vi "sub_dt_fgv.vi"(7 "cmd":enum16{"ini", "dt"}(ring)) -> (3 "dt":u32)   [LabVIEW 2018]
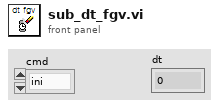
[diagram p1: front panel]
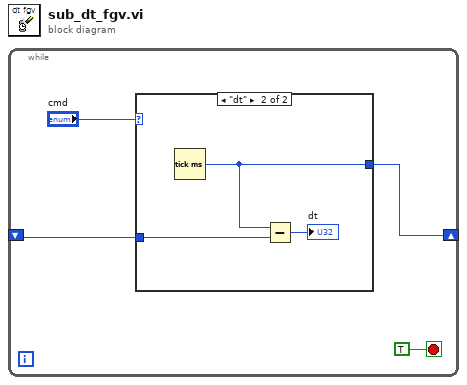
[diagram p0: block diagram]
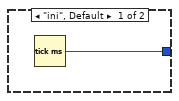
[diagram p2: hidden frame]
diagram:
  n1 = while {
    shift-right: [w1] -> _
    shift-left: _ -> [w2]
    stop <- TRUE stop-if-true
    n2 = case shown="\"dt\"" "cmd" {
      tunnel: w2 -> [_ w8]
      tunnel: [w5 w7] -> w1
      frame "ini", Default {
        n3 = Tick Count (ms)() -> (millisecond timer value=w5:u32)
      }
      frame "dt" {
        n4 = Tick Count (ms)() -> (millisecond timer value=w7:u32)
        n5 = Subtract(x=w7, y=w8) -> (x-y=→"dt":u32)
      }
    }
  }
